vi "NMT.vi"() -> ()   [LabVIEW 2014]
uses:
  <vilib>/CANopenLib/CANOPEN.llb/CANopen Interface Close.vi
panel:
  in  "NMT command":u16(ring)=1 items=["start remote node"=1, "stop remote node"=2, "enter pre-operational"=128, "reset node"=129, "reset communication"=130]
  in  "error in (no error)":errorcluster
  out "error out":errorcluster
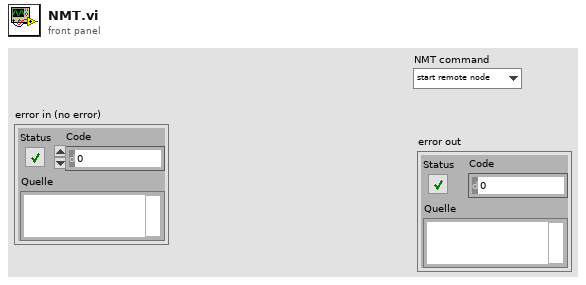
[diagram p1: front panel]
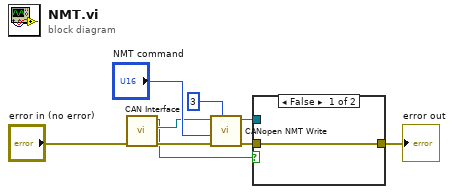
[diagram p0: block diagram]
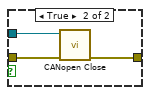
[diagram p2: hidden frame]
diagram:
  n1 = call "CAN Interface.vi"("error in (no error)"="error in (no error)") -> ("error out"=w5:errorcluster, "interface object out"=w4:refnum<k20>, "Interface schließen?"=w1:bool)  [unwired: 8 in]
  n2 = call <vilib>:"CANopen NMT Write.vi"("node-ID (0)"=u8 3 ("node-ID"), "error in (no error)"=w5, "command"="NMT command", "interface object in"=w4) -> ("error out"=w2:errorcluster, "interface object out"=w3:refnum<k20>)  [unwired: 6 in]
  n3 = case shown="False" w1 {
    tunnel: w3 -> [_ w13]
    tunnel: w2 -> [w10 w12]
    tunnel: [w10 w11] -> w9
    frame False {
    }
    frame True {
      n4 = call-poly <vilib>:"CANopen Close.vi"("error in (no error)"=w12, "interface object in"=w13) -> ("error out"=w11:errorcluster)  [unwired: 9 in]
    }
  }
  "error out" <- w9
